vi "Count Down.vi"(8 "error in (no error)":errorcluster, 11 "Worker in":refnum<class "Worker.lvclass">) -> (0 "error out":errorcluster, 3 "Worker out":refnum<class "Worker.lvclass">)   [LabVIEW 2024, in "Worker.lvlib" / "Worker.lvclass"]
uses:
  Worker.lvclass
  C:/Program Files/National Instruments/LabVIEW 2024/vi.lib/ActorFramework/Actor/Actor.lvclass
  Worker Messages/Count Down by One Msg/Count Down by One Msg.lvclass
  C:/Program Files/National Instruments/LabVIEW 2024/vi.lib/ActorFramework/Message/Message.lvclass
  <vilib>/ActorFramework/Actor/Actor.lvclass/Actor.ctl
  <vilib>/ActorFramework/Message Enqueuer/Message Enqueuer.lvclass/Message Enqueuer.ctl
  Worker.lvclass/Worker.ctl
  <vilib>/ActorFramework/Message Enqueuer/Init from Existing Queue.vi
  <vilib>/ActorFramework/Message Enqueuer/Message Enqueuer.lvclass
  <vilib>/ActorFramework/Actor/Actor.lvclass
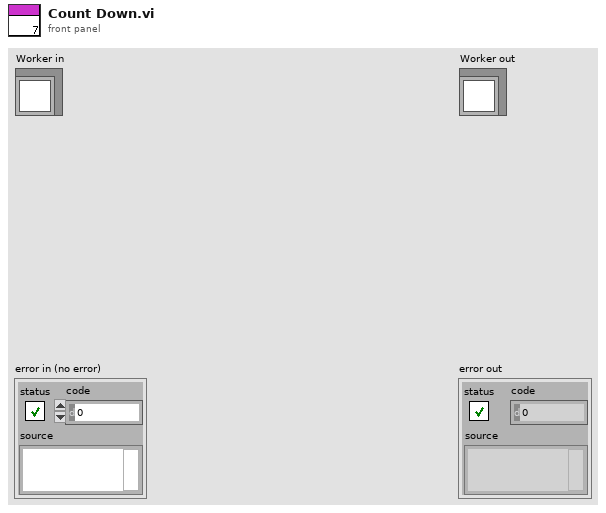
[diagram p1: front panel]
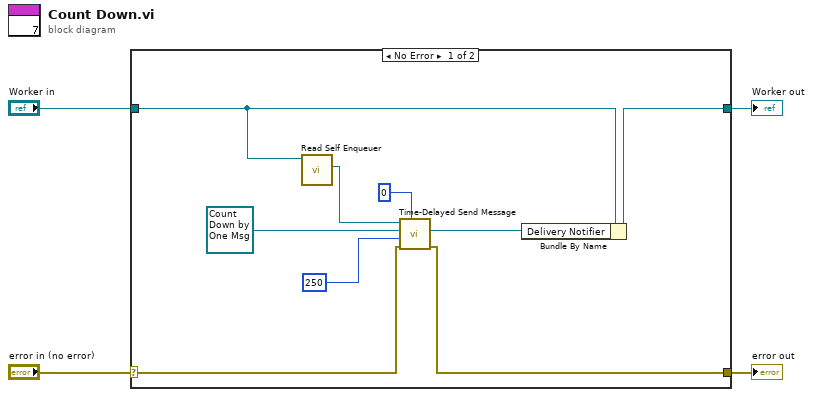
[diagram p0: block diagram]
diagram:
  n1 = case shown="No Error" "error in (no error)" {
    selector: "error in (no error)" -> [w11 w15]
    tunnel: [w10 w15] -> w3
    tunnel: [w8 w14] -> w1
    tunnel: "Worker in" -> [w13 w14]
    frame No Error {
      n2 = call <vilib>:"Read Self Enqueuer.vi"("Actor"=w13) -> ("Self Enqueuer"=w12:refnum<class "Message Enqueuer.lvclass">)  [unwired: 10 in]
      n3 = call <vilib>:"Time-Delayed Send Message.vi"("# Copies (0 = infinite repeat)"=u32 0, "error in (no error)"=w11, "Milliseconds To Wait"=250, "Message"=refnum<class "Count Down by One Msg.lvclass"> refnum ("Worker.lvlib:Count Down by One Msg.lvclass"), "Message Enqueuer"=w12) -> ("error out"=w10:errorcluster, "Delivery Notifier"=w7:refnum<notifier>)  [unwired: 5 in]
      n4 = Bundle By Name(cluster=w13, "Delivery Notifier"=w7) -> (w8:refnum<class "Worker.lvclass">)
    }
    frame Error {
    }
  }
  "error out" <- w3
  "Worker out" <- w1
